vi "algo.run.HostTests.vi"() -> (3 "All Passed?":bool)   [LabVIEW 2022 SP3]
panel:
  in  "error in":errorcluster
  out "error out":errorcluster
  out "Results.out":T1
  in  "filter(s)":string[](array[string])=["hostTests"]
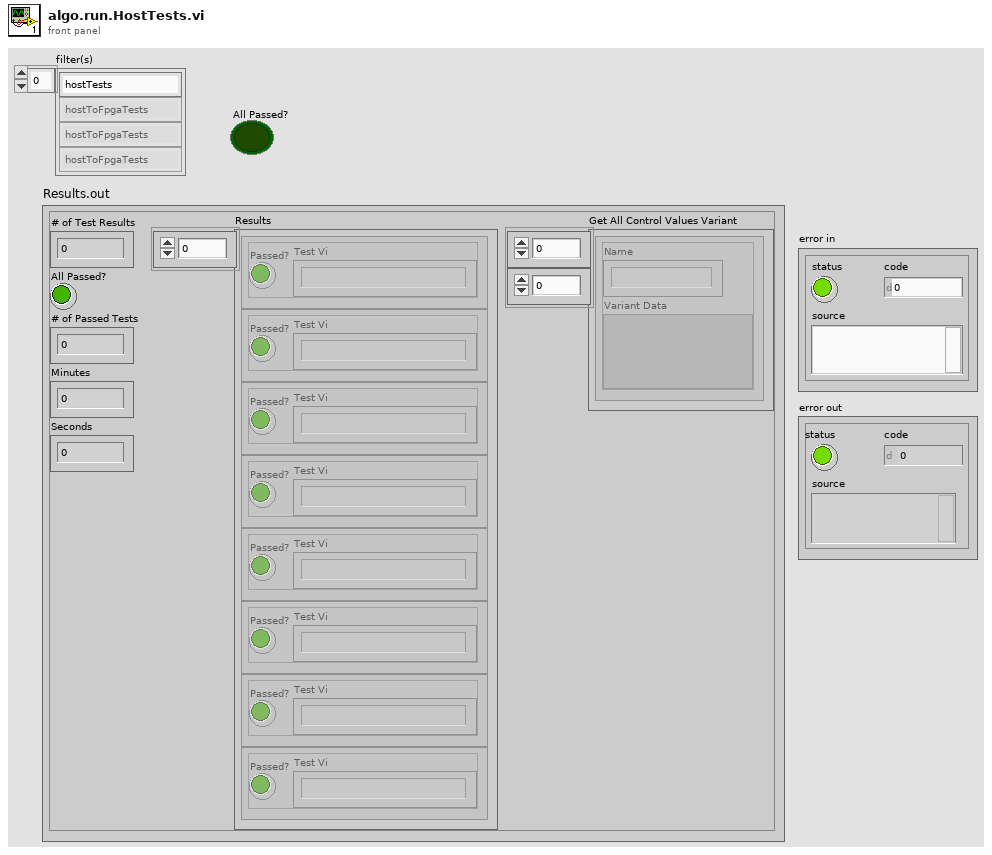
[diagram p1: front panel]
types:
  T1 = cluster{"Results":cluster{"Test Vi":string, "Passed?":bool}[], "# of Test Results":i32, "All Passed?":bool, "# of Passed Tests":i32, "Minutes":u32, "Seconds":u32, "Get All Control Values Variant":cluster{"Name":string, "Variant Data":variant}[][]}
  T2 = cluster{"filter(s)":string[], "path":path, "error in":errorcluster}
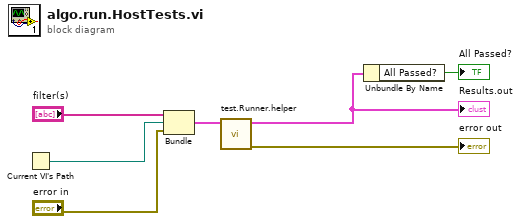
[diagram p0: block diagram]
diagram:
  n1 = Current VI's Path() -> (path=w6:path)
  n2 = Bundle("filter(s)"="filter(s)", "path"=w6, "error in"="error in") -> (w5:T2)  [unwired: 1 in]
  n3 = call "test.Runner.helper.vi"("Parameters.in"=w5) -> ("error out"=→"error out":errorcluster, "Results.out"=w2:T1)  [unwired: 9 in]
  "Results.out" <- w2
  n4 = Unbundle By Name(w2) -> ("All Passed?"=→"All Passed?":bool)
